vi "G2131-i通讯参数 (子VI).vi"() -> (1 "12CO2(dry）":string, 2 "Delta2Min":string, 3 "12CO2":string, 4 "Delta5Min":string, 5 "H2O":string, 6 "13CO2":string, 7 "13CO2（dry）":string)   [LabVIEW 2016]
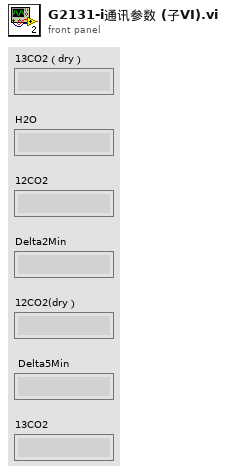
[diagram p1: front panel]
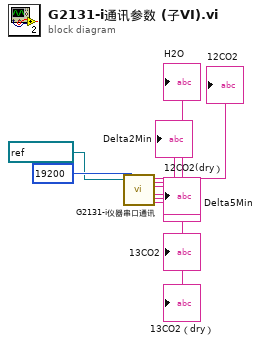
[diagram p0: block diagram]
diagram:
  n1 = call "G2131-i仪器串口通讯.vi"("VISA resource name"=refnum<visa-resource-name> "COM2", "baud rate (9600)"=u32 19200) -> ("Delta2Min"=→"Delta2Min":string, "H2O"=→"H2O":string, "12CO2"=→"12CO2":string, "12CO2(dry）"=→"12CO2(dry）":string, "Delta5Min"=→"Delta5Min":string, "13CO2"=→"13CO2":string, "13CO2（dry）"=→"13CO2（dry）":string)  [unwired: 2 in]
